vi "SLSC Get SLSC Chassis Address.vi"(8 "error in (no error)":errorcluster, 11 "Parent Ref":T1 format="%.0x") -> (0 "error out":errorcluster, 2 "ChassisIDType":i32(ring) items=["ChassisName", "HostnameIPAddress"], 3 "IP Address":string)   [LabVIEW 2017]
uses:
  <vilib>/NI Veristand/Custom Device API/Custom Device Item Ref.ctl
  NationalInstruments.VeriStand.SystemDefinitionAPI
  <vilib>/NI VeriStand/Custom Device API/Custom Device API.lvlib
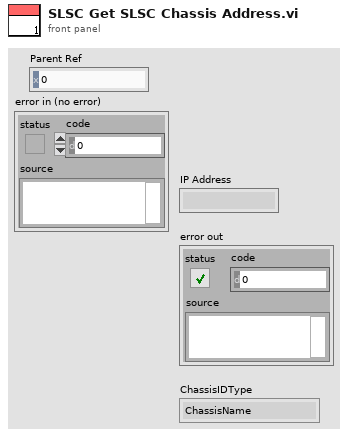
[diagram p1: front panel]
types:
  T1 = typedef "Custom Device API.lvlib/Custom Device Item Ref.ctl" = u64
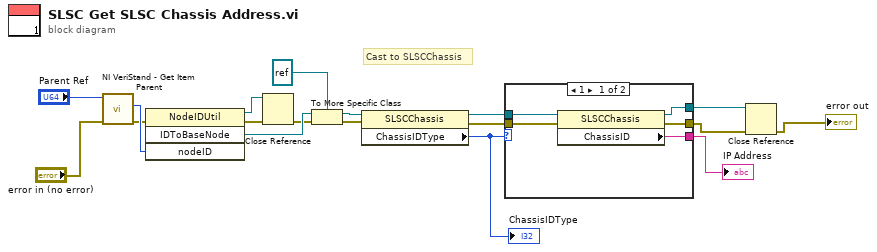
[diagram p0: block diagram]
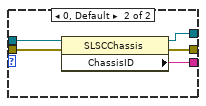
[diagram p2: hidden frame]
diagram:
  # "Cast to SLSCChassis"
  n1 = call <vilib>:"NI VeriStand - Get Item Parent.vi"("error in (no error)"="error in (no error)", "Item Ref in"="Parent Ref") -> ("error out"=w16:errorcluster, "Parent Ref"=w18:T1)  [unwired: 6 in, 2 out]
  n2 = invoke class="NodeIDUtil" method="IDToBaseNode"(error in=w16, "nodeID"=w18) -> (reference out=w10:refnum<k24>, error out=w11:errorcluster, "IDToBaseNode"=w13:refnum<k24>)  [unwired: 2 in, 1 out]
  n3 = Close Reference(reference=w10, error in (no error)=w11) -> (error out=w12:errorcluster)
  n4 = To More Specific Class(target class=refnum<k24> refnum, reference=w13, error in=w12) -> (specific class reference=w7:refnum<k24>, error out=w6:errorcluster)
  n5 = property class="SLSCChassis"(reference=w7, error in=w6) -> (reference out=w5:refnum<k24>, error out=w4:errorcluster, "ChassisIDType"=w1:i32)
  "ChassisIDType" <- w1
  n6 = case shown="1" w1 {
    tunnel: [w23 w28] -> w15
    tunnel: w5 -> [w22 w27]
    tunnel: w4 -> [w21 w26]
    tunnel: [w20 w25] -> w3
    tunnel: [w19 w24] -> w2
    frame 1 {
      n7 = property class="SLSCChassis"(reference=w22, error in=w21) -> (reference out=w20:refnum<k24>, error out=w19:errorcluster, "ChassisID"=w23:string)
    }
    frame 0, Default {
      n8 = property class="SLSCChassis"(reference=w27, error in=w26) -> (reference out=w25:refnum<k24>, error out=w24:errorcluster, "ChassisID"=w28:string)
    }
  }
  "IP Address" <- w15
  n9 = Close Reference(reference=w3, error in (no error)=w2) -> (error out=→"error out":errorcluster)
